vi "GeoData.vi"() -> ()   [LabVIEW 2017] (continued)
OK\tGarvin County\tH1\n73052\t40049\tLindsay\tOK\tGarvin County\tH1\n73075\t40049\tPauls valley\tOK\tGarvin County\tH1\n73074\t40049\tPaoli\tOK\tGarvin County\tH1\n73444\t40049\tHennepin\tOK\tGarvin County\tH1\n73433\t40049\tElmore city\tOK\tGarvin County\tH1\n74872\t40049\tStratford\tOK\tGarvin County\tH1\n73057\t40049\tMaysville\tOK\tGarvin County\tH1\n73095\t40049\tWayne\tOK\tGarvin County\tH1\n73434\t40049\tFoster\tOK\tGarvin County\tH1\n74831\t40049\tByars\tOK\tGarvin County\tH1\n73488\t40049\tTussy\tOK\tGarvin County\tH1\n74865\t40049\tRoff\tOK\tGarvin County\tH1\n73030\t40049\tDavis\tOK\tGarvin County\tH1\n73011\t40049\tBradley\tOK\tGarvin County\tH1\n73010\t40051\tBlanchard\tOK\tGrady County\tH1\n73017\t40051\tCement\tOK\tGrady County\tH1\n73067\t40051\tNinnekah\tOK\tGrady County\tH1\n73065\t40051\tNewcastle\tOK\tGrady County\tH1\n73047\t40051\tHinton\tOK\tGrady County\tH1\n73052\t40051\tLindsay\tOK\tGrady County\tH1\n73079\t40051\tPocasset\tOK\tGrady County\tH1\n73005\t40051\tAnadarko\tOK\tGrady County\tH1\n73004\t40051\tAmber\tOK\tGrady County\tH1\n73018\t40051\tChickasha\tOK\tGrady County\tH1\n73059\t40051\tMinco\tOK\tGrady County\tH1\n73089\t40051\tTuttle\tOK\tGrady County\tH1\n73082\t40051\tRush springs\tOK\tGrady County\tH1\n73092\t40051\tVerden\tOK\tGrady County\tH1\n73055\t40051\tMarlow\tOK\tGrady County\tH1\n73023\t40051\tChickasha\tOK\tGrady County\tH1\n73002\t40051\tAlex\tOK\tGrady County\tH1\n73011\t40051\tBradley\tOK\tGrady County\tH1\n73761\t40053\tNash\tOK\tGrant County\tH1\n74636\t40053\tDeer creek\tOK\tGrant County\tH1\n74643\t40053\tLamont\tOK\tGrant County\tH1\n73759\t40053\tMedford\tOK\tGrant County\tH1\n73771\t40053\tWakita\tOK\tGrant County\tH1\n73766\t40053\tPond creek\tOK\tGrant County\tH1\n74646\t40053\tNardin\tOK\tGrant County\tH1\n74640\t40053\tHunter\tOK\tGrant County\tH1\n73758\t40053\tManchester\tOK\tGrant County\tH1\n73547\t40055\tGranite\tOK\tGreer County\tH1\n73554\t40055\tMangum\tOK\tGreer County\tH1\n73526\t40055\tBlair\tOK\tGreer County\tH1\n73655\t40055\tLone wolf\tOK\tGreer County\tH1\n73673\t40055\tWillow\tOK\tGreer County\tH1\n73554\t40057\tMangum\tOK\tHarmon County\tH1\n73537\t40057\tEldorado\tOK\tHarmon County\tH1\n73544\t40057\tGould\tOK\tHarmon County\tH1\n73550\t40057\tHollis\tOK\tHarmon County\tH1\n73571\t40057\tVinson\tOK\tHarmon County\tH1\n73851\t40059\tMay\tOK\tHarper County\tH1\n73834\t40059\tBuffalo\tOK\tHarper County\tH1\n73855\t40059\tRosston\tOK\tHarper County\tH1\n73848\t40059\tLaverne\tOK\tHarper County\tH1\n74462\t40061\tStigler\tOK\tHaskell County\tH1\n74432\t40061\tEufaula\tOK\tHaskell County\tH1\n74472\t40061\tWhitefield\tOK\tHaskell County\tH1\n74552\t40061\tKinta\tOK\tHaskell County\tH1\n74941\t40061\tKeota\tOK\tHaskell County\tH1\n74944\t40061\tMccurtain\tOK\tHaskell County\tH1\n74561\t40061\tQuinton\tOK\tHaskell County\tH1\n74943\t40061\tLequire\tOK\tHaskell County\tH1\n74570\t40063\tStuart\tOK\tHughes County\tH1\n74531\t40063\tCalvin\tOK\tHughes County\tH1\n74827\t40063\tAtwood\tOK\tHughes County\tH1\n74850\t40063\tLamar\tOK\tHughes County\tH1\n74839\t40063\tDustin\tOK\tHughes County\tH1\n74884\t40063\tWewoka\tOK\tHughes County\tH1\n74848\t40063\tHoldenville\tOK\tHughes County\tH1\n74883\t40063\tWetumka\tOK\tHughes County\tH1\n74825\t40063\tAllen\tOK\tHughes County\tH1\n73532\t40065\tDuke\tOK\tJackson County\tH1\n73521\t40065\tAltus\tOK\tJackson County\tH1\n73537\t40065\tEldorado\tOK\tJackson County\tH1\n73526\t40065\tBlair\tOK\tJackson County\tH1\n73522\t40065\tAltus\tOK\tJackson County\tH1\n73556\t40065\tMartha\tOK\tJackson County\tH1\n73549\t40065\tHeadrick\tOK\tJackson County\tH1\n73560\t40065\tOlustee\tOK\tJackson County\tH1\n73523\t40065\tAltus afb\tOK\tJackson County\tH1\n73539\t40065\tElmer\tOK\tJackson County\tH1\n73520\t40067\tAddington\tOK\tJefferson County\tH1\n73456\t40067\tRingling\tOK\tJefferson County\tH1\n73573\t40067\tWaurika\tOK\tJefferson County\tH1\n73569\t40067\tTerral\tOK\tJefferson County\tH1\n73565\t40067\tRyan\tOK\tJefferson County\tH1\n73548\t40067\tHastings\tOK\tJefferson County\tH1\n74748\t40069\tKenefic\tOK\tJohnston County\tH1\n73447\t40069\tMannsville\tOK\tJohnston County\tH1\n74836\t40069\tConnerville\tOK\tJohnston County\tH1\n73446\t40069\tMadill\tOK\tJohnston County\tH1\n73455\t40069\tRavia\tOK\tJohnston County\tH1\n73461\t40069\tWapanucka\tOK\tJohnston County\tH1\n73432\t40069\tColeman\tOK\tJohnston County\tH1\n73460\t40069\tTishomingo\tOK\tJohnston County\tH1\n73450\t40069\tMilburn\tOK\tJohnston County\tH1\n74525\t40069\tAtoka\tOK\tJohnston County\tH1\n74871\t40069\tStonewall\tOK\tJohnston County\tH1\n74530\t40069\tBromide\tOK\tJohnston County\tH1\n73401\t40069\tArdmore\tOK\tJohnston County\tH1\n73086\t40069\tSulphur\tOK\tJohnston County\tH1\n74820\t40069\tAda\tOK\tJohnston County\tH1\n74856\t40069\tMill creek\tOK\tJohnston County\tH1\n74653\t40071\tTonkawa\tOK\tKay County\tH1\n74631\t40071\tBlackwell\tOK\tKay County\tH1\n74632\t40071\tBraman\tOK\tKay County\tH1\n74604\t40071\tPonca city\tOK\tKay County\tH1\n74652\t40071\tShidler\tOK\tKay County\tH1\n74643\t40071\tLamont\tOK\tKay County\tH1\n74641\t40071\tKaw city\tOK\tKay County\tH1\n74630\t40071\tBillings\tOK\tKay County\tH1\n74646\t40071\tNardin\tOK\tKay County\tH1\n74644\t40071\tMarland\tOK\tKay County\tH1\n74647\t40071\tNewkirk\tOK\tKay County\tH1\n74601\t40071\tPonca city\tOK\tKay County\tH1\n74602\t40071\tPonca city\tOK\tKay County\tH1\n73750\t40073\tKingfisher\tOK\tKingfisher County\tH1\n73762\t40073\tOkarche\tOK\tKingfisher County\tH1\n73742\t40073\tHennessey\tOK\tKingfisher County\tH1\n73734\t40073\tDover\tOK\tKingfisher County\tH1\n73028\t40073\tCrescent\tOK\tKingfisher County\tH1\n73756\t40073\tLoyal\tOK\tKingfisher County\tH1\n73016\t40073\tCashion\tOK\tKingfisher County\tH1\n73764\t40073\tOmega\tOK\tKingfisher County\tH1\n73651\t40075\tHobart\tOK\tKiowa County\tH1\n73041\t40075\tGotebo\tOK\tKiowa County\tH1\n73566\t40075\tSnyder\tOK\tKiowa County\tH1\n73564\t40075\tRoosevelt\tOK\tKiowa County\tH1\n73655\t40075\tLone wolf\tOK\tKiowa County\tH1\n73062\t40075\tMountain view\tOK\tKiowa County\tH1\n73559\t40075\tMountain park\tOK\tKiowa County\tH1\n74547\t40077\tHartshorne\tOK\tLatimer County\tH1\n74563\t40077\tRed oak\tOK\tLatimer County\tH1\n74536\t40077\tClayton\tOK\tLatimer County\tH1\n74559\t40077\tPanola\tOK\tLatimer County\tH1\n74574\t40077\tTuskahoma\tOK\tLatimer County\tH1\n74966\t40077\tWister\tOK\tLatimer County\tH1\n74545\t40077\tGowen\tOK\tLatimer County\tH1\n74571\t40077\tTalihina\tOK\tLatimer County\tH1\n74578\t40077\tWilburton\tOK\tLatimer County\tH1\n74956\t40079\tShady point\tOK\tLe Flore County\tH1\n74957\t40079\tSmithville\tOK\tLe Flore County\tH1\n74577\t40079\tWhitesboro\tOK\tLe Flore County\tH1\n74942\t40079\tLeflore\tOK\tLe Flore County\tH1\n74902\t40079\tPocola\tOK\tLe Flore County\tH1\n74932\t40079\tCameron\tOK\tLe Flore County\tH1\n74935\t40079\tFanshawe\tOK\tLe Flore County\tH1\n74563\t40079\tRed oak\tOK\tLe Flore County\tH1\n74941\t40079\tKeota\tOK\tLe Flore County\tH1\n74549\t40079\tHonobia\tOK\tLe Flore County\tH1\n74947\t40079\tMonroe\tOK\tLe Flore County\tH1\n74953\t40079\tPoteau\tOK\tLe Flore County\tH1\n74959\t40079\tSpiro\tOK\tLe Flore County\tH1\n74939\t40079\tHodgen\tOK\tLe Flore County\tH1\n74930\t40079\tBokoshe\tOK\tLe Flore County\tH1\n74944\t40079\tMccurtain\tOK\tLe Flore County\tH1\n74966\t40079\tWister\tOK\tLe Flore County\tH1\n74571\t40079\tTalihina\tOK\tLe Flore County\tH1\n74940\t40079\tHowe\tOK\tLe Flore County\tH1\n74937\t40079\tHeavener\tOK\tLe Flore County\tH1\n74901\t40079\tArkoma\tOK\tLe Flore County\tH1\n74949\t40079\tMuse\tOK\tLe Flore County\tH1\n74951\t40079\tPanama\tOK\tLe Flore County\tH1\n74834\t40081\tChandler\tOK\tLincoln County\tH1\n74832\t40081\tCarney\tOK\tLincoln County\tH1\n74875\t40081\tTryon\tOK\tLincoln County\tH1\n74881\t40081\tWellston\tOK\tLincoln County\tH1\n74855\t40081\tMeeker\tOK\tLincoln County\tH1\n74824\t40081\tAgra\tOK\tLincoln County\tH1\n74026\t40081\tDavenport\tOK\tLincoln County\tH1\n74079\t40081\tStroud\tOK\tLincoln County\tH1\n74869\t40081\tSparks\tOK\tLincoln County\tH1\n73054\t40081\tLuther\tOK\tLincoln County\tH1\n74023\t40081\tCushing\tOK\tLincoln County\tH1\n74059\t40081\tPerkins\tOK\tLincoln County\tH1\n74851\t40081\tMcloud\tOK\tLincoln County\tH1\n74028\t40081\tDepew\tOK\tLincoln County\tH1\n73045\t40081\tHarrah\tOK\tLincoln County\tH1\n74864\t40081\tPrague\tOK\tLincoln County\tH1\n73073\t40083\tOrlando\tOK\tLogan County\tH1\n73063\t40083\tMulhall\tOK\tLogan County\tH1\n73044\t40083\tGuthrie\tOK\tLogan County\tH1\n74881\t40083\tWellston\tOK\tLogan County\tH1\n73028\t40083\tCrescent\tOK\tLogan County\tH1\n73056\t40083\tMarshall\tOK\tLogan County\tH1\n73027\t40083\tCoyle\tOK\tLogan County\tH1\n73054\t40083\tLuther\tOK\tLogan County\tH1\n73025\t40083\tEdmond\tOK\tLogan County\tH1\n74059\t40083\tPerkins\tOK\tLogan County\tH1\n73050\t40083\tLangston\tOK\tLogan County\tH1\n73034\t40083\tEdmond\tOK\tLogan County\tH1\n73016\t40083\tCashion\tOK\tLogan County\tH1\n73058\t40083\tMeridian\tOK\tLogan County\tH1\n73007\t40083\tArcadia\tOK\tLogan County\tH1\n73430\t40085\tBurneyville\tOK\tLove County\tH1\n73441\t40085\tLeon\tOK\tLove County\tH1\n73456\t40085\tRingling\tOK\tLove County\tH1\n73463\t40085\tWilson\tOK\tLove County\tH1\n73448\t40085\tMarietta\tOK\tLove County\tH1\n73453\t40085\tOverbrook\tOK\tLove County\tH1\n73459\t40085\tThackerville\tOK\tLove County\tH1\n73401\t40085\tArdmore\tOK\tLove County\tH1\n73010\t40087\tBlanchard\tOK\tMcClain County\tH1\n73065\t40087\tNewcastle\tOK\tMcClain County\tH1\n73052\t40087\tLindsay\tOK\tMcClain County\tH1\n73074\t40087\tPaoli\tOK\tMcClain County\tH1\n74872\t40087\tStratford\tOK\tMcClain County\tH1\n73057\t40087\tMaysville\tOK\tMcClain County\tH1\n73095\t40087\tWayne\tOK\tMcClain County\tH1\n73080\t40087\tPurcell\tOK\tMcClain County\tH1\n74831\t40087\tByars\tOK\tMcClain County\tH1\n73072\t40087\tNorman\tOK\tMcClain County\tH1\n73093\t40087\tWashington\tOK\tMcClain County\tH1\n73002\t40087\tAlex\tOK\tMcClain County\tH1\n73031\t40087\tDibble\tOK\tMcClain County\tH1\n74957\t40089\tSmithville\tOK\tMcCurtain County\tH1\n74766\t40089\tWright city\tOK\tMcCurtain County\tH1\n74754\t40089\tRingold\tOK\tMcCurtain County\tH1\n74724\t40089\tBethel\tOK\tMcCurtain County\tH1\n74728\t40089\tBroken bow\tOK\tMcCurtain County\tH1\n74745\t40089\tIdabel\tOK\tMcCurtain County\tH1\n74963\t40089\tWatson\tOK\tMcCurtain County\tH1\n74755\t40089\tRufe\tOK\tMcCurtain County\tH1\n74750\t40089\tMillerton\tOK\tMcCurtain County\tH1\n74752\t40089\tPickens\tOK\tMcCurtain County\tH1\n74562\t40089\tRattan\tOK\tMcCurtain County\tH1\n74734\t40089\tEagletown\tOK\tMcCurtain County\tH1\n74740\t40089\tHaworth\tOK\tMcCurtain County\tH1\n74736\t40089\tGarvin\tOK\tMcCurtain County\tH1\n74764\t40089\tValliant\tOK\tMcCurtain County\tH1\n74722\t40089\tBattiest\tOK\tMcCurtain County\tH1\n74737\t40089\tGolden\tOK\tMcCurtain County\tH1\n74428\t40091\tCouncil hill\tOK\tMcIntosh County\tH1\n74438\t40091\tHitchita\tOK\tMcIntosh County\tH1\n74432\t40091\tEufaula\tOK\tMcIntosh County\tH1\n74455\t40091\tPorum\tOK\tMcIntosh County\tH1\n74450\t40091\tOktaha\tOK\tMcIntosh County\tH1\n74426\t40091\tChecotah\tOK\tMcIntosh County\tH1\n74845\t40091\tHanna\tOK\tMcIntosh County\tH1\n74459\t40091\tRentiesville\tOK\tMcIntosh County\tH1\n74445\t40091\tMorris\tOK\tMcIntosh County\tH1\n74437\t40091\tHenryetta\tOK\tMcIntosh County\tH1\n74469\t40091\tWarner\tOK\tMcIntosh County\tH1\n73760\t40093\tMeno\tOK\tMajor County\tH1\n73747\t40093\tIsabella\tOK\tMajor County\tH1\n73718\t40093\tAmes\tOK\tMajor County\tH1\n73754\t40093\tLahoma\tOK\tMajor County\tH1\n73729\t40093\tCleo springs\tOK\tMajor County\tH1\n73768\t40093\tRingwood\tOK\tMajor County\tH1\n73838\t40093\tChester\tOK\tMajor County\tH1\n73737\t40093\tFairview\tOK\tMajor County\tH1\n73726\t40093\tCarmen\tOK\tMajor County\tH1\n73447\t40095\tMannsville\tOK\tMarshall County\tH1\n73446\t40095\tMadill\tOK\tMarshall County\tH1\n73439\t40095\tKingston\tOK\tMarshall County\tH1\n73448\t40095\tMarietta\tOK\tMarshall County\tH1\n73440\t40095\tLebanon\tOK\tMarshall County\tH1\n73401\t40095\tArdmore\tOK\tMarshall County\tH1\n74036\t40097\tInola\tOK\tMayes County\tH1\n74366\t40097\tSpavinaw\tOK\tMayes County\tH1\n74441\t40097\tHulbert\tOK\tMayes County\tH1\n74019\t40097\tClaremore\tOK\tMayes County\tH1\n74361\t40097\tPryor\tOK\tMayes County\tH1\n74332\t40097\tBig cabin\tOK\tMayes County\tH1\n74367\t40097\tStrang\tOK\tMayes County\tH1\n74337\t40097\tChouteau\tOK\tMayes County\tH1\n74364\t40097\tRose\tOK\tMayes County\tH1\n74352\t40097\tLocust grove\tOK\tMayes County\tH1\n74452\t40097\tPeggs\tOK\tMayes County\tH1\n74330\t40097\tAdair\tOK\tMayes County\tH1\n74340\t40097\tDisney\tOK\tMayes County\tH1\n74016\t40097\tChelsea\tOK\tMayes County\tH1\n74301\t40097\tVinita\tOK\tMayes County\tH1\n74365\t40097\tSalina\tOK\tMayes County\tH1\n74350\t40097\tLangley\tOK\tMayes County\tH1\n73098\t40099\tWynnewood\tOK\tMurray County\tH1\n73444\t40099\tHennepin\tOK\tMurray County\tH1\n73032\t40099\tDougherty\tOK\tMurray County\tH1\n74865\t40099\tRoff\tOK\tMurray County\tH1\n73030\t40099\tDavis\tOK\tMurray County\tH1\n73086\t40099\tSulphur\tOK\tMurray County\tH1\n74856\t40099\tMill creek\tOK\tMurray County\tH1\n74403\t40101\tMuskogee\tOK\tMuskogee County\tH1\n74428\t40101\tCouncil hill\tOK\tMuskogee County\tH1\n74434\t40101\tFort gibson\tOK\tMuskogee County\tH1\n74422\t40101\tBoynton\tOK\tMuskogee County\tH1\n74423\t40101\tBraggs\tOK\tMuskogee County\tH1\n74402\t40101\tMuskogee\tOK\tMuskogee County\tH1\n74468\t40101\tWainwright\tOK\tMuskogee County\tH1\n74455\t40101\tPorum\tOK\tMuskogee County\tH1\n74463\t40101\tTaft\tOK\tMuskogee County\tH1\n74450\t40101\tOktaha\tOK\tMuskogee County\tH1\n74401\t40101\tMuskogee\tOK\tMuskogee County\tH1\n74435\t40101\tGore\tOK\tMuskogee County\tH1\n74445\t40101\tMorris\tOK\tMuskogee County\tH1\n74436\t40101\tHaskell\tOK\tMuskogee County\tH1\n74470\t40101\tWebbers falls\tOK\tMuskogee County\tH1\n74469\t40101\tWarner\tOK\tMuskogee County\tH1\n73073\t40103\tOrlando\tOK\tNoble County\tH1\n73757\t40103\tLucien\tOK\tNoble County\tH1\n73061\t40103\tMorrison\tOK\tNoble County\tH1\n73077\t40103\tPerry\tOK\tNoble County\tH1\n74651\t40103\tRed rock\tOK\tNoble County\tH1\n74032\t40103\tGlencoe\tOK\tNoble County\tH1\n74075\t40103\tStillwater\tOK\tNoble County\tH1\n74630\t40103\tBillings\tOK\tNoble County\tH1\n74644\t40103\tMarland\tOK\tNoble County\tH1\n74601\t40103\tPonca city\tOK\tNoble County\tH1\n74027\t40105\tDelaware\tOK\tNowata County\tH1\n74042\t40105\tLenapah\tOK\tNowata County\tH1\n74048\t40105\tNowata\tOK\tNowata County\tH1\n74006\t40105\tBartlesville\tOK\tNowata County\tH1\n74083\t40105\tWann\tOK\tNowata County\tH1\n74016\t40105\tChelsea\tOK\tNowata County\tH1\n74072\t40105\tS coffeyville\tOK\tNowata County\tH1\n74301\t40105\tVinita\tOK\tNowata County\tH1\n74010\t40107\tBristow\tOK\tOkfuskee County\tH1\n74880\t40107\tWeleetka\tOK\tOkfuskee County\tH1\n74447\t40107\tOkmulgee\tOK\tOkfuskee County\tH1\n74860\t40107\tPaden\tOK\tOkfuskee County\tH1\n74833\t40107\tCastle\tOK\tOkfuskee County\tH1\n74829\t40107\tBoley\tOK\tOkfuskee County\tH1\n74883\t40107\tWetumka\tOK\tOkfuskee County\tH1\n74859\t40107\tOkemah\tOK\tOkfuskee County\tH1\n74864\t40107\tPrague\tOK\tOkfuskee County\tH1\n73012\t40109\tEdmond\tOK\tOklahoma County\tH1\n73013\t40109\tEdmond\tOK\tOklahoma County\tH1\n73121\t40109\tOklahoma city\tOK\tOklahoma County\tH1\n73099\t40109\tYukon\tOK\tOklahoma County\tH1\n73127\t40109\tOklahoma city\tOK\tOklahoma County\tH1\n73128\t40109\tOklahoma city\tOK\tOklahoma County\tH1\n73109\t40109\tOklahoma city\tOK\tOklahoma County\tH1\n73129\t40109\tOklahoma city\tOK\tOklahoma County\tH1\n73150\t40109\tOklahoma city\tOK\tOklahoma County\tH1\n73111\t40109\tOklahoma city\tOK\tOklahoma County\tH1\n73003\t40109\tEdmond\tOK\tOklahoma County\tH1\n74857\t40109\tNewalla\tOK\tOklahoma County\tH1\n73194\t40109\tOklahoma city\tOK\tOklahoma County\tH1\n73065\t40109\tNewcastle\tOK\tOklahoma County\tH1\n73179\t40109\tOklahoma city\tOK\tOklahoma County\tH1\n73165\t40109\tOklahoma city\tOK\tOklahoma County\tH1\n73122\t40109\tOklahoma city\tOK\tOklahoma County\tH1\n73108\t40109\tOklahoma city\tOK\tOklahoma County\tH1\n73103\t40109\tOklahoma city\tOK\tOklahoma County\tH1\n73131\t40109\tOklahoma city\tOK\tOklahoma County\tH1\n73140\t40109\tOklahoma city\tOK\tOklahoma County\tH1\n73184\t40109\tOklahoma city\tOK\tOklahoma County\tH1\n73078\t40109\tPiedmont\tOK\tOklahoma County\tH1\n73118\t40109\tOklahoma city\tOK\tOklahoma County\tH1\n73105\t40109\tOklahoma city\tOK\tOklahoma County\tH1\n73132\t40109\tOklahoma city\tOK\tOklahoma County\tH1\n73157\t40109\tOklahoma city\tOK\tOklahoma County\tH1\n73101\t40109\tOklahoma city\tOK\tOklahoma County\tH1\n73151\t40109\tOklahoma city\tOK\tOklahoma County\tH1\n73195\t40109\tOklahoma city\tOK\tOklahoma County\tH1\n73049\t40109\tJones\tOK\tOklahoma County\tH1\n73169\t40109\tOklahoma city\tOK\tOklahoma County\tH1\n73110\t40109\tOklahoma city\tOK\tOklahoma County\tH1\n73112\t40109\tOklahoma city\tOK\tOklahoma County\tH1\n73116\t40109\tOklahoma city\tOK\tOklahoma County\tH1\n73139\t40109\tOklahoma city\tOK\tOklahoma County\tH1\n73083\t40109\tEdmond\tOK\tOklahoma County\tH1\n73141\t40109\tOklahoma city\tOK\tOklahoma County\tH1\n73156\t40109\tOklahoma city\tOK\tOklahoma County\tH1\n73152\t40109\tOklahoma city\tOK\tOklahoma County\tH1\n73054\t40109\tLuther\tOK\tOklahoma County\tH1\n73162\t40109\tOklahoma city\tOK\tOklahoma County\tH1\n73119\t40109\tOklahoma city\tOK\tOklahoma County\tH1\n73149\t40109\tOklahoma city\tOK\tOklahoma County\tH1\n73008\t40109\tBethany\tOK\tOklahoma County\tH1\n73113\t40109\tOklahoma city\tOK\tOklahoma County\tH1\n73155\t40109\tOklahoma city\tOK\tOklahoma County\tH1\n73144\t40109\tOklahoma city\tOK\tOklahoma County\tH1\n73097\t40109\tWheatland\tOK\tOklahoma County\tH1\n73066\t40109\tNicoma park\tOK\tOklahoma County\tH1\n73025\t40109\tEdmond\tOK\tOklahoma County\tH1\n73160\t40109\tOklahoma city\tOK\tOklahoma County\tH1\n73115\t40109\tOklahoma city\tOK\tOklahoma County\tH1\n73120\t40109\tOklahoma city\tOK\tOklahoma County\tH1\n73107\t40109\tOklahoma city\tOK\tOklahoma County\tH1\n73084\t40109\tSpencer\tOK\tOklahoma County\tH1\n73123\t40109\tOklahoma city\tOK\tOklahoma County\tH1\n73130\t40109\tOklahoma city\tOK\tOklahoma County\tH1\n74851\t40109\tMcloud\tOK\tOklahoma County\tH1\n73172\t40109\tOklahoma city\tOK\tOklahoma County\tH1\n73143\t40109\tOklahoma city\tOK\tOklahoma County\tH1\n73125\t40109\tOklahoma city\tOK\tOklahoma County\tH1\n73034\t40109\tEdmond\tOK\tOklahoma County\tH1\n73117\t40109\tOklahoma city\tOK\tOklahoma County\tH1\n73135\t40109\tOklahoma city\tOK\tOklahoma County\tH1\n73145\t40109\tOklahoma city\tOK\tOklahoma County\tH1\n73146\t40109\tOklahoma city\tOK\tOklahoma County\tH1\n73134\t40109\tOklahoma city\tOK\tOklahoma County\tH1\n73007\t40109\tArcadia\tOK\tOklahoma County\tH1\n73137\t40109\tOklahoma city\tOK\tOklahoma County\tH1\n73045\t40109\tHarrah\tOK\tOklahoma County\tH1\n73020\t40109\tChoctaw\tOK\tOklahoma County\tH1\n73104\t40109\tOklahoma city\tOK\tOklahoma County\tH1\n73106\t40109\tOklahoma city\tOK\tOklahoma County\tH1\n73159\t40109\tOklahoma city\tOK\tOklahoma County\tH1\n73102\t40109\tOklahoma city\tOK\tOklahoma County\tH1\n73114\t40109\tOklahoma city\tOK\tOklahoma County\tH1\n73142\t40109\tOklahoma city\tOK\tOklahoma County\tH1\n73147\t40109\tOklahoma city\tOK\tOklahoma County\tH1\n73136\t40109\tOklahoma city\tOK\tOklahoma County\tH1\n73154\t40109\tOklahoma city\tOK\tOklahoma County\tH1\n73148\t40109\tOklahoma city\tOK\tOklahoma County\tH1\n73190\t40109\tOklahoma city\tOK\tOklahoma County\tH1\n74421\t40111\tBeggs\tOK\tOkmulgee County\tH1\n74428\t40111\tCouncil hill\tOK\tOkmulgee County\tH1\n74422\t40111\tBoynton\tOK\tOkmulgee County\tH1\n74880\t40111\tWeleetka\tOK\tOkmulgee County\tH1\n74047\t40111\tMounds\tOK\tOkmulgee County\tH1\n74431\t40111\tDewar\tOK\tOkmulgee County\tH1\n74445\t40111\tMorris\tOK\tOkmulgee County\tH1\n74447\t40111\tOkmulgee\tOK\tOkmulgee County\tH1\n74436\t40111\tHaskell\tOK\tOkmulgee County\tH1\n74460\t40111\tSchulter\tOK\tOkmulgee County\tH1\n74437\t40111\tHenryetta\tOK\tOkmulgee County\tH1\n74456\t40111\tPreston\tOK\tOkmulgee County\tH1\n74103\t40113\tTulsa\tOK\tOsage County\tH1\n74051\t40113\tOchelata\tOK\tOsage County\tH1\n74115\t40113\tTulsa\tOK\tOsage County\tH1\n74035\t40113\tHominy\tOK\tOsage County\tH1\n74061\t40113\tRamona\tOK\tOsage County\tH1\n74022\t40113\tCopan\tOK\tOsage County\tH1\n74633\t40113\tBurbank\tOK\tOsage County\tH1\n74073\t40113\tSperry\tOK\tOsage County\tH1\n74126\t40113\tTulsa\tOK\tOsage County\tH1\n74650\t40113\tRalston\tOK\tOsage County\tH1\n74604\t40113\tPonca city\tOK\tOsage County\tH1\n74652\t40113\tShidler\tOK\tOsage County\tH1\n74070\t40113\tSkiatook\tOK\tOsage County\tH1\n74056\t40113\tPawhuska\tOK\tOsage County\tH1\n74637\t40113\tFairfax\tOK\tOsage County\tH1\n74002\t40113\tBarnsdall\tOK\tOsage County\tH1\n74063\t40113\tSand springs\tOK\tOsage County\tH1\n74054\t40113\tOsage\tOK\tOsage County\tH1\n74001\t40113\tAvant\tOK\tOsage County\tH1\n74003\t40113\tBartlesville\tOK\tOsage County\tH1\n74127\t40113\tTulsa\tOK\tOsage County\tH1\n74106\t40113\tTulsa\tOK\tOsage County\tH1\n74084\t40113\tWynona\tOK\tOsage County\tH1\n74060\t40113\tPrue\tOK\tOsage County\tH1\n74370\t40115\tWyandotte\tOK\tOttawa County\tH1\n74339\t40115\tCommerce\tOK\tOttawa County\tH1\n74358\t40115\tNorth miami\tOK\tOttawa County\tH1\n74333\t40115\tBluejacket\tOK\tOttawa County\tH1\n74360\t40115\tPicher\tOK\tOttawa County\tH1\n74331\t40115\tAfton\tOK\tOttawa County\tH1\n74354\t40115\tMiami\tOK\tOttawa County\tH1\n74363\t40115\tQuapaw\tOK\tOttawa County\tH1\n74335\t40115\tCardin\tOK\tOttawa County\tH1\n74344\t40115\tGrove\tOK\tOttawa County\tH1\n74343\t40115\tFairland\tOK\tOttawa County\tH1\n74045\t40117\tMaramec\tOK\tPawnee County\tH1\n73061\t40117\tMorrison\tOK\tPawnee County\tH1\n74038\t40117\tJennings\tOK\tPawnee County\tH1\n74650\t40117\tRalston\tOK\tPawnee County\tH1\n74020\t40117\tCleveland\tOK\tPawnee County\tH1\n74032\t40117\tGlencoe\tOK\tPawnee County\tH1\n74644\t40117\tMarland\tOK\tPawnee County\tH1\n74044\t40117\tMannford\tOK\tPawnee County\tH1\n74081\t40117\tTerlton\tOK\tPawnee County\tH1\n74058\t40117\tPawnee\tOK\tPawnee County\tH1\n74034\t40117\tHallett\tOK\tPawnee County\tH1\n74045\t40119\tMaramec\tOK\tPayne County\tH1\n73073\t40119\tOrlando\tOK\tPayne County\tH1\n73063\t40119\tMulhall\tOK\tPayne County\tH1\n74824\t40119\tAgra\tOK\tPayne County\tH1\n74076\t40119\tStillwater\tOK\tPayne County\tH1\n73077\t40119\tPerry\tOK\tPayne County\tH1\n74030\t40119\tDrumright\tOK\tPayne County\tH1\n74085\t40119\tYale\tOK\tPayne County\tH1\n73027\t40119\tCoyle\tOK\tPayne County\tH1\n74023\t40119\tCushing\tOK\tPayne County\tH1\n74032\t40119\tGlencoe\tOK\tPayne County\tH1\n74075\t40119\tStillwater\tOK\tPayne County\tH1\n74059\t40119\tPerkins\tOK\tPayne County\tH1\n74062\t40119\tRipley\tOK\tPayne County\tH1\n74077\t40119\tStillwater\tOK\tPayne County\tH1\n74078\t40119\tStillwater\tOK\tPayne County\tH1\n74074\t40119\tStillwater\tOK\tPayne County\tH1\n74442\t40121\tIndianola\tOK\tPittsburg County\tH1\n74553\t40121\tKiowa\tOK\tPittsburg County\tH1\n74547\t40121\tHartshorne\tOK\tPittsburg County\tH1\n74554\t40121\tKrebs\tOK\tPittsburg County\tH1\n74425\t40121\tCanadian\tOK\tPittsburg County\tH1\n74570\t40121\tStuart\tOK\tPittsburg County\tH1\n74529\t40121\tBlocker\tOK\tPittsburg County\tH1\n74462\t40121\tStigler\tOK\tPittsburg County\tH1\n74430\t40121\tCrowder\tOK\tPittsburg County\tH1\n74522\t40121\tAlderson\tOK\tPittsburg County\tH1\n74432\t40121\tEufaula\tOK\tPittsburg County\tH1\n74536\t40121\tClayton\tOK\tPittsburg County\tH1\n74565\t40121\tSavanna\tOK\tPittsburg County\tH1\n74552\t40121\tKinta\tOK\tPittsburg County\tH1\n74501\t40121\tMcalester\tOK\tPittsburg County\tH1\n74576\t40121\tWardville\tOK\tPittsburg County\tH1\n74546\t40121\tHaileyville\tOK\tPittsburg County\tH1\n74528\t40121\tBlanco\tOK\tPittsburg County\tH1\n74561\t40121\tQuinton\tOK\tPittsburg County\tH1\n74560\t40121\tPittsburg\tOK\tPittsburg County\tH1\n74578\t40121\tWilburton\tOK\tPittsburg County\tH1\n74572\t40123\tTupelo\tOK\tPontotoc County\tH1\n74842\t40123\tFittstown\tOK\tPontotoc County\tH1\n74872\t40123\tStratford\tOK\tPontotoc County\tH1\n74821\t40123\tAda\tOK\tPontotoc County\tH1\n74831\t40123\tByars\tOK\tPontotoc County\tH1\n74871\t40123\tStonewall\tOK\tPontotoc County\tH1\n74865\t40123\tRoff\tOK\tPontotoc County\tH1\n74844\t40123\tFrancis\tOK\tPontotoc County\tH1\n74820\t40123\tAda\tOK\tPontotoc County\tH1\n74843\t40123\tFitzhugh\tOK\tPontotoc County\tH1\n74825\t40123\tAllen\tOK\tPontotoc County\tH1\n74801\t40125\tShawnee\tOK\tPottawatomie County\tH1\n74857\t40125\tNewalla\tOK\tPottawatomie County\tH1\n74878\t40125\tWanette\tOK\tPottawatomie County\tH1\n74855\t40125\tMeeker\tOK\tPottawatomie County\tH1\n74849\t40125\tKonawa\tOK\tPottawatomie County\tH1\n74079\t40125\tStroud\tOK\tPottawatomie County\tH1\n74873\t40125\tTecumseh\tOK\tPottawatomie County\tH1\n74802\t40125\tShawnee\tOK\tPottawatomie County\tH1\n74866\t40125\tSaint louis\tOK\tPottawatomie County\tH1\n74804\t40125\tShawnee\tOK\tPottawatomie County\tH1\n73051\t40125\tLexington\tOK\tPottawatomie County\tH1\n74851\t40125\tMcloud\tOK\tPottawatomie County\tH1\n74854\t40125\tMaud\tOK\tPottawatomie County\tH1\n74826\t40125\tAsher\tOK\tPottawatomie County\tH1\n74852\t40125\tMacomb\tOK\tPottawatomie County\tH1\n73045\t40125\tHarrah\tOK\tPottawatomie County\tH1\n74840\t40125\tEarlsboro\tOK\tPottawatomie County\tH1\n74864\t40125\tPrague\tOK\tPottawatomie County\tH1\n74735\t40127\tFort towson\tOK\tPushmataha County\tH1\n74754\t40127\tRingold\tOK\tPushmataha County\tH1\n74558\t40127\tNashoba\tOK\tPushmataha County\tH1\n74536\t40127\tClayton\tOK\tPushmataha County\tH1\n74574\t40127\tTuskahoma\tOK\tPushmataha County\tH1\n74557\t40127\tMoyers\tOK\tPushmataha County\tH1\n74543\t40127\tFinley\tOK\tPushmataha County\tH1\n74567\t40127\tSnow\tOK\tPushmataha County\tH1\n74523\t40127\tAntlers\tOK\tPushmataha County\tH1\n74562\t40127\tRattan\tOK\tPushmataha County\tH1\n74571\t40127\tTalihina\tOK\tPushmataha County\tH1\n74521\t40127\tAlbion\tOK\tPushmataha County\tH1\n73660\t40129\tReydon\tOK\tRoger Mills County\tH1\n73644\t40129\tElk city\tOK\tRoger Mills County\tH1\n73662\t40129\tSayre\tOK\tRoger Mills County\tH1\n73666\t40129\tSweetwater\tOK\tRoger Mills County\tH1\n73650\t40129\tHammon\tOK\tRoger Mills County\tH1\n73628\t40129\tCheyenne\tOK\tRoger Mills County\tH1\n73638\t40129\tCrawford\tOK\tRoger Mills County\tH1\n73625\t40129\tButler\tOK\tRoger Mills County\tH1\n73654\t40129\tLeedey\tOK\tRoger Mills County\tH1\n73642\t40129\tDurham\tOK\tRoger Mills County\tH1\n74036\t40131\tInola\tOK\tRogers County\tH1\n74053\t40131\tOologah\tOK\tRogers County\tH1\n74017\t40131\tClaremore\tOK\tRogers County\tH1\n74021\t40131\tCollinsville\tOK\tRogers County\tH1\n74031\t40131\tFoyil\tOK\tRogers County\tH1\n74048\t40131\tNowata\tOK\tRogers County\tH1\n74116\t40131\tTulsa\tOK\tRogers County\tH1\n74015\t40131\tCatoosa\tOK\tRogers County\tH1\n74019\t40131\tClaremore\tOK\tRogers County\tH1\n74080\t40131\tTalala\tOK\tRogers County\tH1\n74361\t40131\tPryor\tOK\tRogers County\tH1\n74332\t40131\tBig cabin\tOK\tRogers County\tH1\n74055\t40131\tOwasso\tOK\tRogers County\tH1\n74018\t40131\tClaremore\tOK\tRogers County\tH1\n74016\t40131\tChelsea\tOK\tRogers County\tH1\n74849\t40133\tKonawa\tOK\tSeminole County\tH1\n74884\t40133\tWewoka\tOK\tSeminole County\tH1\n74867\t40133\tSasakwa\tOK\tSeminole County\tH1\n74804\t40133\tShawnee\tOK\tSeminole County\tH1\n74837\t40133\tCromwell\tOK\tSeminole County\tH1\n74854\t40133\tMaud\tOK\tSeminole County\tH1\n74830\t40133\tBowlegs\tOK\tSeminole County\tH1\n74848\t40133\tHoldenville\tOK\tSeminole County\tH1\n74859\t40133\tOkemah\tOK\tSeminole County\tH1\n74868\t40133\tSeminole\tOK\tSeminole County\tH1\n74840\t40133\tEarlsboro\tOK\tSeminole County\tH1\n74955\t40135\tSallisaw\tOK\tSequoyah County\tH1\n74962\t40135\tVian\tOK\tSequoyah County\tH1\n74936\t40135\tGans\tOK\tSequoyah County\tH1\n74945\t40135\tMarble city\tOK\tSequoyah County\tH1\n74946\t40135\tMoffett\tOK\tSequoyah County\tH1\n74435\t40135\tGore\tOK\tSequoyah County\tH1\n74948\t40135\tMuldrow\tOK\tSequoyah County\tH1\n74931\t40135\tBunch\tOK\tSequoyah County\tH1\n74954\t40135\tRoland\tOK\tSequoyah County\tH1\n73529\t40137\tComanche\tOK\tStephens County\tH1\n73491\t40137\tVelma\tOK\tStephens County\tH1\n73425\t40137\tCountyline\tOK\tStephens County\tH1\n73533\t40137\tDuncan\tOK\tStephens County\tH1\n73055\t40137\tMarlow\tOK\tStephens County\tH1\n73442\t40137\tLoco\tOK\tStephens County\tH1\n73951\t40139\tTyrone\tOK\tTexas County\tH1\n73939\t40139\tGoodwell\tOK\tTexas County\tH1\n73944\t40139\tHardesty\tOK\tTexas County\tH1\n73901\t40139\tAdams\tOK\tTexas County\tH1\n73942\t40139\tGuymon\tOK\tTexas County\tH1\n73945\t40139\tHooker\tOK\tTexas County\tH1\n73949\t40139\tTexhoma\tOK\tTexas County\tH1\n73570\t40141\tTipton\tOK\tTillman County\tH1\n73553\t40141\tLoveland\tOK\tTillman County\tH1\n73566\t40141\tSnyder\tOK\tTillman County\tH1\n73552\t40141\tIndiahoma\tOK\tTillman County\tH1\n73551\t40141\tHollister\tOK\tTillman County\tH1\n73555\t40141\tManitou\tOK\tTillman County\tH1\n73528\t40141\tChattanooga\tOK\tTillman County\tH1\n73546\t40141\tGrandfield\tOK\tTillman County\tH1\n73530\t40141\tDavidson\tOK\tTillman County\tH1\n73542\t40141\tFrederick\tOK\tTillman County\tH1\n74066\t40143\tSapulpa\tOK\tTulsa County\tH1\n74103\t40143\tTulsa\tOK\tTulsa County\tH1\n74129\t40143\tTulsa\tOK\tTulsa County\tH1\n74115\t40143\tTulsa\tOK\tTulsa County\tH1\n74145\t40143\tTulsa\tOK\tTulsa County\tH1\n74159\t40143\tTulsa\tOK\tTulsa County\tH1\n74155\t40143\tTulsa\tOK\tTulsa County\tH1\n74149\t40143\tTulsa\tOK\tTulsa County\tH1\n74153\t40143\tTulsa\tOK\tTulsa County\tH1\n74171\t40143\tTulsa\tOK\tTulsa County\tH1\n74012\t40143\tBroken arrow\tOK\tTulsa County\tH1\n74033\t40143\tGlenpool\tOK\tTulsa County\tH1\n74053\t40143\tOologah\tOK\tTulsa County\tH1\n74128\t40143\tTulsa\tOK\tTulsa County\tH1\n74114\t40143\tTulsa\tOK\tTulsa County\tH1\n74132\t40143\tTulsa\tOK\tTulsa County\tH1\n74150\t40143\tTulsa\tOK\tTulsa County\tH1\n74141\t40143\tTulsa\tOK\tTulsa County\tH1\n74008\t40143\tBixby\tOK\tTulsa County\tH1\n74021\t40143\tCollinsville\tOK\tTulsa County\tH1\n74037\t40143\tJenks\tOK\tTulsa County\tH1\n74073\t40143\tSperry\tOK\tTulsa County\tH1\n74126\t40143\tTulsa\tOK\tTulsa County\tH1\n74116\t40143\tTulsa\tOK\tTulsa County\tH1\n74120\t40143\tTulsa\tOK\tTulsa County\tH1\n74135\t40143\tTulsa\tOK\tTulsa County\tH1\n74172\t40143\tTulsa\tOK\tTulsa County\tH1\n74013\t40143\tBroken arrow\tOK\tTulsa County\tH1\n74015\t40143\tCatoosa\tOK\tTulsa County\tH1\n74137\t40143\tTulsa\tOK\tTulsa County\tH1\n74170\t40143\tTulsa\tOK\tTulsa County\tH1\n74131\t40143\tTulsa\tOK\tTulsa County\tH1\n74152\t40143\tTulsa\tOK\tTulsa County\tH1\n74182\t40143\tTulsa\tOK\tTulsa County\tH1\n74193\t40143\tTulsa\tOK\tTulsa County\tH1\n74104\t40143\tTulsa\tOK\tTulsa County\tH1\n74070\t40143\tSkiatook\tOK\tTulsa County\tH1\n74108\t40143\tTulsa\tOK\tTulsa County\tH1\n74047\t40143\tMounds\tOK\tTulsa County\tH1\n74055\t40143\tOwasso\tOK\tTulsa County\tH1\n74148\t40143\tTulsa\tOK\tTulsa County\tH1\n74192\t40143\tTulsa\tOK\tTulsa County\tH1\n74186\t40143\tTulsa\tOK\tTulsa County\tH1\n74105\t40143\tTulsa\tOK\tTulsa County\tH1\n74107\t40143\tTulsa\tOK\tTulsa County\tH1\n74112\t40143\tTulsa\tOK\tTulsa County\tH1\n74130\t40143\tTulsa\tOK\tTulsa County\tH1\n74146\t40143\tTulsa\tOK\tTulsa County\tH1\n74157\t40143\tTulsa\tOK\tTulsa County\tH1\n74043\t40143\tLeonard\tOK\tTulsa County\tH1\n74011\t40143\tBroken arrow\tOK\tTulsa County\tH1\n74063\t40143\tSand springs\tOK\tTulsa County\tH1\n74044\t40143\tMannford\tOK\tTulsa County\tH1\n74050\t40143\tOakhurst\tOK\tTulsa County\tH1\n74110\t40143\tTulsa\tOK\tTulsa County\tH1\n74117\t40143\tTulsa\tOK\tTulsa County\tH1\n74436\t40143\tHaskell\tOK\tTulsa County\tH1\n74101\t40143\tTulsa\tOK\tTulsa County\tH1\n74169\t40143\tTulsa\tOK\tTulsa County\tH1\n74147\t40143\tTulsa\tOK\tTulsa County\tH1\n74158\t40143\tTulsa\tOK\tTulsa County\tH1\n74156\t40143\tTulsa\tOK\tTulsa County\tH1\n74014\t40143\tBroken arrow\tOK\tTulsa County\tH1\n74127\t40143\tTulsa\tOK\tTulsa County\tH1\n74106\t40143\tTulsa\tOK\tTulsa County\tH1\n74133\t40143\tTulsa\tOK\tTulsa County\tH1\n74119\t40143\tTulsa\tOK\tTulsa County\tH1\n74136\t40143\tTulsa\tOK\tTulsa County\tH1\n74134\t40143\tTulsa\tOK\tTulsa County\tH1\n74187\t40143\tTulsa\tOK\tTulsa County\tH1\n74403\t40145\tMuskogee\tOK\tWagoner County\tH1\n74429\t40145\tCoweta\tOK\tWagoner County\tH1\n74036\t40145\tInola\tOK\tWagoner County\tH1\n74434\t40145\tFort gibson\tOK\tWagoner County\tH1\n74454\t40145\tPorter\tOK\tWagoner County\tH1\n74458\t40145\tRedbird\tOK\tWagoner County\tH1\n74008\t40145\tBixby\tOK\tWagoner County\tH1\n74116\t40145\tTulsa\tOK\tWagoner County\tH1\n74015\t40145\tCatoosa\tOK\tWagoner County\tH1\n74108\t40145\tTulsa\tOK\tWagoner County\tH1\n74337\t40145\tChouteau\tOK\tWagoner County\tH1\n74352\t40145\tLocust grove\tOK\tWagoner County\tH1\n74436\t40145\tHaskell\tOK\tWagoner County\tH1\n74446\t40145\tOkay\tOK\tWagoner County\tH1\n74014\t40145\tBroken arrow\tOK\tWagoner County\tH1\n74467\t40145\tWagoner\tOK\tWagoner County\tH1\n74029\t40147\tDewey\tOK\tWashington County\tH1\n74051\t40147\tOchelata\tOK\tWashington County\tH1\n74082\t40147\tVera\tOK\tWashington County\tH1\n74061\t40147\tRamona\tOK\tWashington County\tH1\n74005\t40147\tBartlesville\tOK\tWashington County\tH1\n74022\t40147\tCopan\tOK\tWashington County\tH1\n74021\t40147\tCollinsville\tOK\tWashington County\tH1\n74048\t40147\tNowata\tOK\tWashington County\tH1\n74080\t40147\tTalala\tOK\tWashington County\tH1\n74006\t40147\tBartlesville\tOK\tWashington County\tH1\n74070\t40147\tSkiatook\tOK\tWashington County\tH1\n74083\t40147\tWann\tOK\tWashington County\tH1\n74003\t40147\tBartlesville\tOK\tWashington County\tH1\n73632\t40149\tCordell\tOK\tWashita County\tH1\n73096\t40149\tWeatherford\tOK\tWashita County\tH1\n73661\t40149\tRocky\tOK\tWashita County\tH1\n73041\t40149\tGotebo\tOK\tWashita County\tH1\n73622\t40149\tBessie\tOK\tWashita County\tH1\n73644\t40149\tElk city\tOK\tWashita County\tH1\n73647\t40149\tFoss\tOK\tWashita County\tH1\n73015\t40149\tCarnegie\tOK\tWashita County\tH1\n73664\t40149\tSentinel\tOK\tWashita County\tH1\n73641\t40149\tDill city\tOK\tWashita County\tH1\n73021\t40149\tColony\tOK\tWashita County\tH1\n73626\t40149\tCanute\tOK\tWashita County\tH1\n73624\t40149\tBurns flat\tOK\tWashita County\tH1\n73024\t40149\tCorn\tOK\tWashita County\tH1\n73601\t40149\tClinton\tOK\tWashita County\tH1\n73062\t40149\tMountain view\tOK\tWashita County\tH1\n73716\t40151\tAline\tOK\tWoods County\tH1\n73860\t40151\tWaynoka\tOK\tWoods County\tH1\n73729\t40151\tCleo springs\tOK\tWoods County\tH1\n73731\t40151\tDacoma\tOK\tWoods County\tH1\n73726\t40151\tCarmen\tOK\tWoods County\tH1\n73746\t40151\tHopeton\tOK\tWoods County\tH1\n73842\t40151\tFreedom\tOK\tWoods County\tH1\n73717\t40151\tAlva\tOK\tWoods County\tH1\n73841\t40153\tFort supply\tOK\tWoodward County\tH1\n73840\t40153\tFargo\tOK\tWoodward County\tH1\n73857\t40153\tSharon\tOK\tWoodward County\tH1\n73801\t40153\tWoodward\tOK\tWoodward County\tH1\n73853\t40153\tMutual\tOK\tWoodward County\tH1\n73852\t40153\tMooreland\tOK\tWoodward County\tH1\n97883\t41001\tUnion\tOR\tBaker County\tH1\n97814\t41001\tBaker city\tOR\tBaker County\tH1\n97833\t41001\tHaines\tOR\tBaker County\tH1\n97905\t41001\tDurkee\tOR\tBaker County\tH1\n97870\t41001\tRichland\tOR\tBaker County\tH1\n97834\t41001\tHalfway\tOR\tBaker County\tH1\n97867\t41001\tNorth powder\tOR\tBaker County\tH1\n97837\t41001\tHereford\tOR\tBaker County\tH1\n97819\t41001\tBridgeport\tOR\tBaker County\tH1\n97877\t41001\tSumpter\tOR\tBaker County\tH1\n97884\t41001\tUnity\tOR\tBaker County\tH1\n97907\t41001\tHuntington\tOR\tBaker County\tH1\n97840\t41001\tOxbow\tOR\tBaker County\tH1\n97330\t41003\tCorvallis\tOR\tBenton County\tH1\n97331\t41003\tCorvallis\tOR\tBenton County\tH1\n97324\t41003\tAlsea\tOR\tBenton County\tH1\n97333\t41003\tCorvallis\tOR\tBenton County\tH1\n97339\t41003\tCorvallis\tOR\tBenton County\tH1\n97448\t41003\tJunction city\tOR\tBenton County\tH1\n97456\t41003\tMonroe\tOR\tBenton County\tH1\n97321\t41003\tAlbany\tOR\tBenton County\tH1\n97361\t41003\tMonmouth\tOR\tBenton County\tH1\n97370\t41003\tPhilomath\tOR\tBenton County\tH1\n97326\t41003\tBlodgett\tOR\tBenton County\tH1\n97140\t41005\tSherwood\tOR\tClackamas County\tH1\n97049\t41005\tRhododendron\tOR\tClackamas County\tH1\n97017\t41005\tColton\tOR\tClackamas County\tH1\n97362\t41005\tMount angel\tOR\tClackamas County\tH1\n97028\t41005\tGovernment camp\tOR\tClackamas County\tH1\n97055\t41005\tSandy\tOR\tClackamas County\tH1\n97038\t41005\tMolalla\tOR\tClackamas County\tH1\n97089\t41005\tDamascus\tOR\tClackamas County\tH1\n97009\t41005\tBoring\tOR\tClackamas County\tH1\n97206\t41005\tPortland\tOR\tClackamas County\tH1\n97375\t41005\tScotts mills\tOR\tClackamas County\tH1\n97062\t41005\tTualatin\tOR\tClackamas County\tH1\n97071\t41005\tWoodburn\tOR\tClackamas County\tH1\n97022\t41005\tEagle creek\tOR\tClackamas County\tH1\n97013\t41005\tCanby\tOR\tClackamas County\tH1\n97004\t41005\tBeavercreek\tOR\tClackamas County\tH1\n97011\t41005\tBrightwood\tOR\tClackamas County\tH1\n97019\t41005\tCorbett\tOR\tClackamas County\tH1\n97086\t41005\tHappy valley\tOR\tClackamas County\tH1\n97269\t41005\tPortland\tOR\tClackamas County\tH1\n97132\t41005\tNewberg\tOR\tClackamas County\tH1\n97219\t41005\tPortland\tOR\tClackamas County\tH1\n97067\t41005\tWelches\tOR\tClackamas County\tH1\n97027\t41005\tGladstone\tOR\tClackamas County\tH1\n97002\t41005\tAurora\tOR\tClackamas County\tH1\n97222\t41005\tPortland\tOR\tClackamas County\tH1\n97045\t41005\tOregon city\tOR\tClackamas County\tH1\n97068\t41005\tWest linn\tOR\tClackamas County\tH1\n97015\t41005\tClackamas\tOR\tClackamas County\tH1\n97023\t41005\tEstacada\tOR\tClackamas County\tH1\n97080\t41005\tGresham\tOR\tClackamas County\tH1\n97042\t41005\tMulino\tOR\tClackamas County\tH1\n97268\t41005\tPortland\tOR\tClackamas County\tH1\n97202\t41005\tPortland\tOR\tClackamas County\tH1\n97267\t41005\tPortland\tOR\tClackamas County\tH1\n97035\t41005\tLake oswego\tOR\tClackamas County\tH1\n97034\t41005\tLake oswego\tOR\tClackamas County\tH1\n97032\t41005\tHubbard\tOR\tClackamas County\tH1\n97070\t41005\tWilsonville\tOR\tClackamas County\tH1\n97036\t41005\tMarylhurst\tOR\tClackamas County\tH1\n97146\t41007\tWarrenton\tOR\tClatsop County\tH1\n97016\t41007\tClatskanie\tOR\tClatsop County\tH1\n97102\t41007\tArch cape\tOR\tClatsop County\tH1\n97145\t41007\tTolovana park\tOR\tClatsop County\tH1\n97138\t41007\tSeaside\tOR\tClatsop County\tH1\n97103\t41007\tAstoria\tOR\tClatsop County\tH1\n97110\t41007\tCannon beach\tOR\tClatsop County\tH1\n97131\t41007\tNehalem\tOR\tClatsop County\tH1\n97121\t41007\tHammond\tOR\tClatsop County\tH1\n97053\t41009\tWarren\tOR\tColumbia County\tH1\n97018\t41009\tColumbia city\tOR\tColumbia County\tH1\n97051\t41009\tSaint helens\tOR\tColumbia County\tH1\n97016\t41009\tClatskanie\tOR\tColumbia County\tH1\n97054\t41009\tDeer island\tOR\tColumbia County\tH1\n97231\t41009\tPortland\tOR\tColumbia County\tH1\n97048\t41009\tRainier\tOR\tColumbia County\tH1\n97056\t41009\tScappoose\tOR\tColumbia County\tH1\n97064\t41009\tVernonia\tOR\tColumbia County\tH1\n97466\t41011\tPowers\tOR\tCoos County\tH1\n97450\t41011\tLanglois\tOR\tCoos County\tH1\n97407\t41011\tAllegany\tOR\tCoos County\tH1\n97414\t41011\tBroadbent\tOR\tCoos County\tH1\n97458\t41011\tMyrtle point\tOR\tCoos County\tH1\n97459\t41011\tNorth bend\tOR\tCoos County\tH1\n97411\t41011\tBandon\tOR\tCoos County\tH1\n97423\t41011\tCoquille\tOR\tCoos County\tH1\n97420\t41011\tCoos bay\tOR\tCoos County\tH1\n97449\t41011\tLakeside\tOR\tCoos County\tH1\n97753\t41013\tPowell butte\tOR\tCrook County\tH1\n97754\t41013\tPrineville\tOR\tCrook County\tH1\n97701\t41013\tBend\tOR\tCrook County\tH1\n97751\t41013\tPaulina\tOR\tCrook County\tH1\n97760\t41013\tTerrebonne\tOR\tCrook County\tH1\n97752\t
